vi "InitTagGroup.vi"(5 "updateInterval":i32=250, 6 "error IO":errorcluster, 7 "Tag List":T1[](array[typedef]), 9 "reference":refnum<k24>) -> (0 "error out":errorcluster, 3 "reference 2":refnum<k24>)   [LabVIEW 2019]
uses:
  <vilib>/NI/Current Value Table/Type Defs/Single Tag.ctl
  <vilib>/NI/Current Value Table/Type Defs/Data Types.ctl
  F:/src/HUTCDLSVN/Machine/CDL0100/TagEngine/LVOPCUA.NET/LVOPC.NETInterface/bin/Release/LVOPC.NETInterface.dll
  LVOPCUA.NET/LVOPC.NETInterface/bin/Release/LVOPC.NETInterface.dll
  <vilib>/NI/Current Value Table/Current Value Table.lvlib
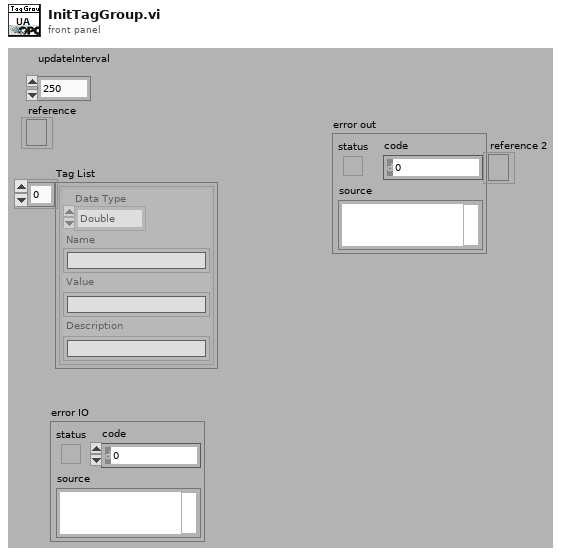
[diagram p1: front panel]
types:
  T1 = typedef "Current Value Table.lvlib/Single Tag.ctl" = cluster{"Data Type":T2, "Name":string, "Value":string, "Description":string}
  T2 = typedef "Current Value Table.lvlib/Data Types.ctl" = enum16{"Double", "Single", "I64", "I32", "I16", "I8", "U64", "U32", "U16", "U8", "String", "Boolean", "Array of U8", "Array of U16", "Array of U32", "Array of U64", "Array of I64", "Array of I32", "Array of I16", "Array of I8", "Array of Double", "Array of Single", "Array of Boolean", "Array of String"}
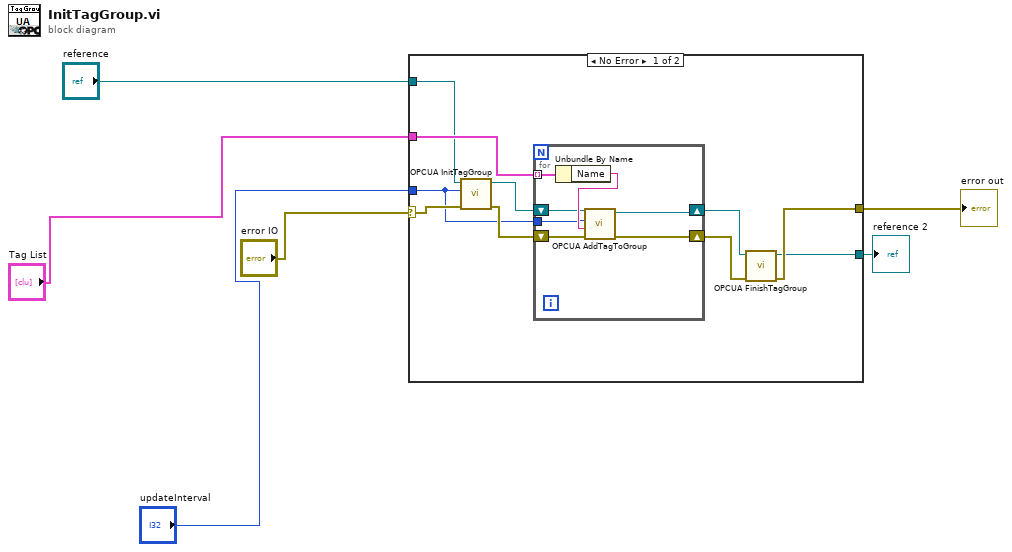
[diagram p0: block diagram]
diagram:
  n1 = case shown="No Error" "error IO" {
    selector: "error IO" -> [w16 w25]
    tunnel: [w13 w25] -> w6
    tunnel: "Tag List" -> [w12 _]
    tunnel: [w11 w24] -> w1
    tunnel: "updateInterval" -> [w7 _]
    tunnel: "reference" -> [w10 w24]
    frame No Error {
      n2 = call "OPCUA InitTagGroup.vi"("error in (no error)"=w16, "publish interval (ms)"=w7, "reference"=w10) -> ("error out"=w15:errorcluster, "reference 2"=w9:refnum<k24>)  [unwired: 7 in]
      n3 = for {
        shift-right: [w22] -> w14
        shift-left: w15 -> [w23]
        tunnel: w12 -> [w21] mode=indexing
        shift-right: [w18] -> w8
        shift-left: w9 -> [w19]
        tunnel: w7 -> [w17]
        n4 = Unbundle By Name(w21) -> ("Name"=w20:string)
        n5 = call "OPCUA AddTagToGroup.vi"("error in (no error)"=w23, "Tag"=w20, "SamplingInterval"=w17, "reference"=w19) -> ("error out"=w22:errorcluster, "reference 2"=w18:refnum<k24>)  [unwired: 6 in]
      }
      n6 = call "OPCUA FinishTagGroup.vi"("error in (no error)"=w14, "reference"=w8) -> ("error out"=w13:errorcluster, "reference 2"=w11:refnum<k24>)  [unwired: 8 in]
    }
    frame Error {
    }
  }
  "error out" <- w6
  "reference 2" <- w1
